vi "SLSC Create Line Properties.vi"(10 "Line Number":i32, 11 "Port Number":i32) -> (3 "Outgoing configuration":T3(array[cluster])=[{"Channel Name"="LED1_Green", "SLSC Name"="Bool.LED1.NI.GreenBool", "Channel"={"Type"=enum."Input", "Units"="", "Default Value"=1.0, "Faultable"=FALSE, "Scalable"=FALSE}, "Enum Names"=["Vsup_Off", "Vsup_0", "Vsup_1"], "Enum Values"=[0, 1, 2]}, {"Channel Name"="Scratchpad8", "SLSC Name"="U32.Scratchpad8.NI.Scratchpad.AsUInt32.U8", "Channel"={"Type"=enum."Input", "Units"="", "Default Value"=12.0, "Faultable"=FALSE, "Scalable"=FALSE}, "Enum Names"=["Vsup_Off", "Vsup_0", "Vsup_1"], "Enum Values"=[0, 1, 2]}])   [LabVIEW 2020, in "SLSC-12201 DIO System Explorer.lvlib"]
uses:
  SLSC-12201 DIO System Explorer.lvlib
  <vilib>/NI VeriStand/Custom Device API/Custom Device Channel.ctl
  <vilib>/NI VeriStand/Custom Device API/Custom Device Channel Type.ctl
  <vilib>/NI VeriStand/Custom Device API/Custom Device API.lvlib
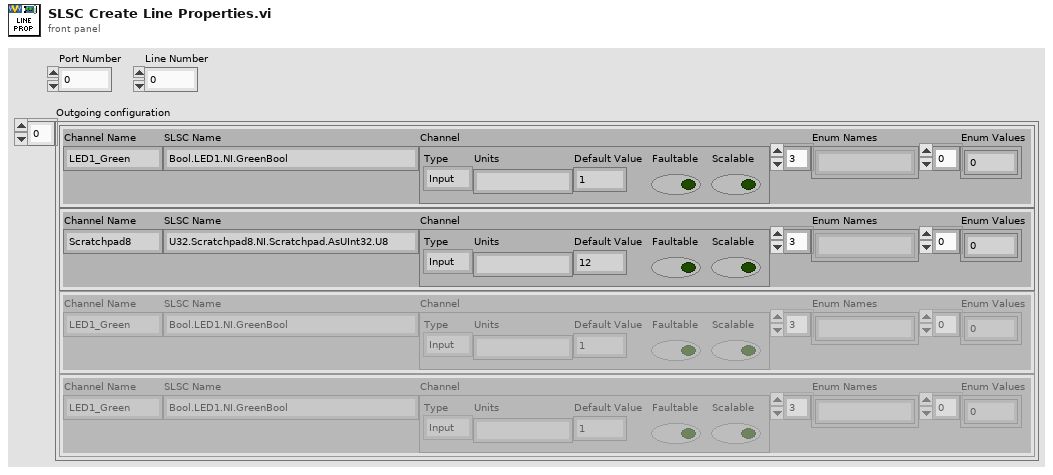
[diagram p1: front panel]
types:
  T1 = typedef "Custom Device API.lvlib/Custom Device Channel.ctl" = cluster{"Type":T2, "Units":string, "Default Value":dbl, "Faultable":bool, "Scalable":bool}
  T2 = typedef "Custom Device API.lvlib/Custom Device Channel Type.ctl" = enum16{"Input", "Output"}
  T3 = cluster{"Channel Name":string, "SLSC Name":string, "Channel":T1, "Enum Names":string[], "Enum Values":i32[]}[]
  T4 = cluster{"Channel Name":string, "SLSC Name":string, "Enum Names":string[], "Enum Values":i32[]}
  T5 = cluster{"Channel Name":string, "SLSC Name":string, "Enum Names":string[], "Enum Values":i32[]}[]
  T6 = cluster{"Channel Name":string, "Channel ":string, "output cluster":T1, "Enum Names":string[], "Enum Values":i32[]}
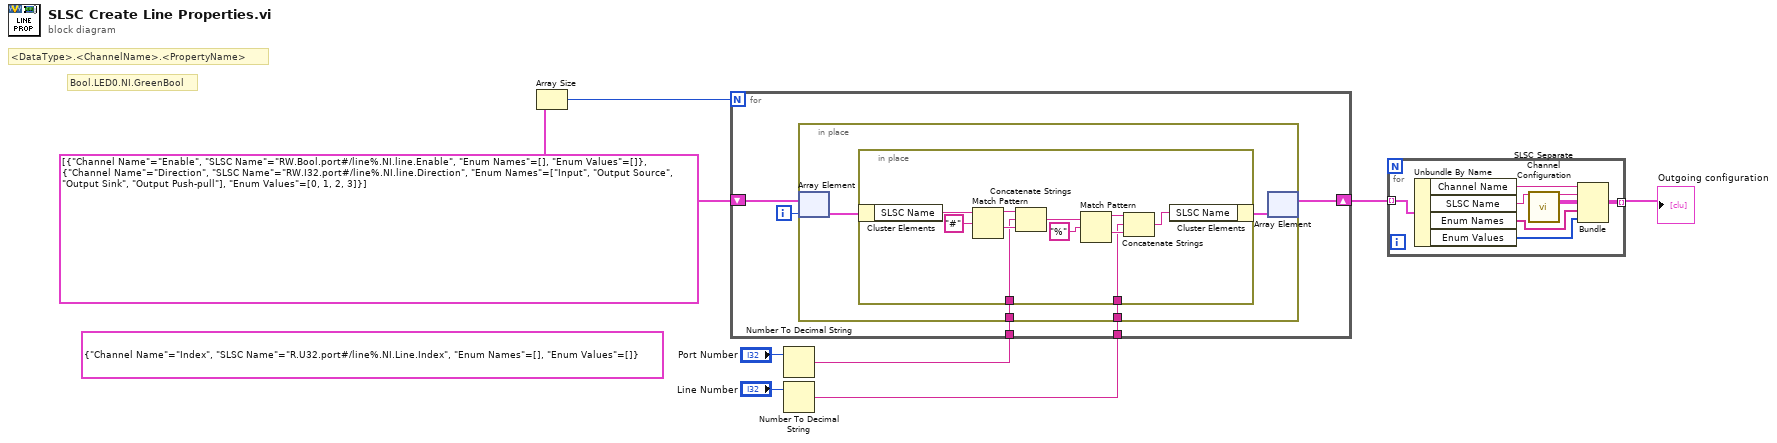
[diagram p0: block diagram]
diagram:
  (unwired) T4 {"Channel Name"="Index", "SLSC Name"="R.U32.port#/line%.NI.Line.Index", "Enum Names"=[], "Enum Values"=[]}
  w1 = T5 [{"Channel Name"="Enable", "SLSC Name"="RW.Bool.port#/line%.NI.line.Enable", "Enum Names"=[], "Enum Values"=[]}, {"Channel Name"="Direction", "SLSC Name"="RW.I32.port#/line%.NI.line.Direction", "Enum Names"=["Input", "Output Source", "Output Sink", "Output Push-pull"], "Enum Values"=[0, 1, 2, 3]}]
  # "Bool.LED0.NI.GreenBool"
  # "<DataType>.<ChannelName>.<PropertyName>"
  n1 = Array Size(array=w1) -> (size(s)=w8:i32)
  n2 = Number To Decimal String(number="Port Number") -> (decimal integer string=w6:string)  [unwired: 1 in]
  n3 = Number To Decimal String(number="Line Number") -> (decimal integer string=w5:string)  [unwired: 1 in]
  n4 = for {
    N: w8 -> [_]
    shift-right: [w12] -> w3
    shift-left: w1 -> [w13]
    tunnel: w6 -> [w10]
    tunnel: w5 -> [w9]
    i -> [w11]
    n5 = in-place {
      in-place-border: w10 -> [w15]
      in-place-border: w9 -> [w14]
      n6 = in-place-array #1(w13, w11) -> (w17:T4)
      n7 = in-place {
        in-place-border: w15 -> [w24]
        in-place-border: w14 -> [w19]
        n8 = in-place-cluster #2(w17) -> ("SLSC Name"=w28:string)
        n9 = Match Pattern(string=w28, regular expression="#") -> (before substring=w26:string, after substring=w25:string)  [unwired: 1 in, 2 out]
        n10 = Concatenate Strings(w26, w24, w25) -> (w20:string)
        n11 = Match Pattern(string=w20, regular expression="%") -> (before substring=w22:string, after substring=w23:string)  [unwired: 1 in, 2 out]
        n12 = Concatenate Strings(w22, w19, w23) -> (w18:string)
        n13 = in-place-cluster #2("SLSC Name"=w18) -> (w16:T4)
      }
      n14 = in-place-array #1(w16) -> (w12:T5)  [unwired: 1 out]
    }
  }
  n15 = for {
    tunnel: w3 -> [w36] mode=indexing
    tunnel: [w31] -> w2 mode=indexing
    n16 = Unbundle By Name(w36) -> ("Channel Name"=w35:string, "SLSC Name"=w34:string, "Enum Names"=w29:string[], "Enum Values"=w30:i32[])
    n17 = call "SLSC Separate Channel Configuration.vi"("Encoded String"=w34) -> ("Channel"=w33:string, "output cluster"=w32:T1)  [unwired: 9 in, 4 out]
    n18 = Bundle("Channel Name"=w35, "Channel"=w33, "output cluster"=w32, "Enum Names"=w29, "Enum Values"=w30) -> (w31:T6)  [unwired: 1 in]
  }
  "Outgoing configuration" <- w2
